vi "Pre Launch Init.vi"(11 "Actor_UI_Template in":refnum<class "Actor_UI_Template.lvclass">) -> (0 "error out":errorcluster, 3 "Actor_UI_Template out":refnum<class "Actor_UI_Template.lvclass">)   [LabVIEW 2020, in "Actor_UI_Template.lvlib" / "Actor_UI_Template.lvclass"]
doc: "(<B>Filename</B>: Actor Framework.lvlib:Actor.lvclass:Pre Launch Init.vi)\n\nDefines behavior that occurs after the Launch Nested Actor method is invoked but before the actor's Actor Core method begins running.\n\nBy default, this method does nothing. A descendant class may override it to define behavior."
uses:
  Actor_UI_Template.lvclass
  Actor_UI_Template.lvclass/Actor_UI_Template.ctl
  <vilib>/ActorFramework/Actor/Actor.lvclass
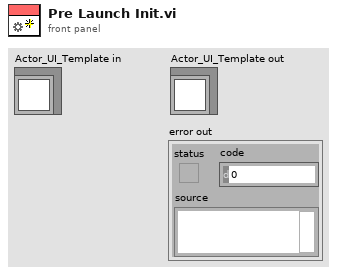
[diagram p1: front panel]
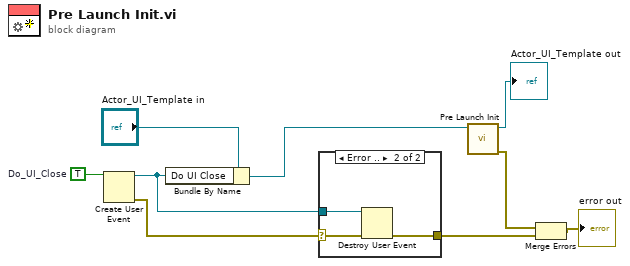
[diagram p0: block diagram]
diagram:
  w8 = TRUE  # Do_UI_Close
  n1 = Create User Event(user event datatype=w8) -> (user event=w4:refnum<user-event>, error out=w5:errorcluster)  [unwired: 1 in]
  n2 = Bundle By Name(cluster="Actor_UI_Template in", "Do UI Close"=w4) -> (w6:refnum<class "Actor_UI_Template.lvclass">)
  n3 = case shown="Error .." w5 {
    selector: w5 -> [w10 w13]
    tunnel: [w10 w12] -> w3
    tunnel: w4 -> [_ w11]
    frame No Error {
    }
    frame Error {
      n4 = Destroy User Event(user event=w11, error in=w13) -> (error out=w12:errorcluster)
    }
  }
  n5 = call-parent "Pre Launch Init.vi"("Actor in"=w6) -> ("error out"=w2:errorcluster, "Actor out"=→"Actor_UI_Template out":refnum<class "Actor_UI_Template.lvclass">)  [unwired: 9 in]
  n6 = Merge Errors(w2, w3) -> (→"error out":errorcluster)
